vi "SUbvi double counter.vi"   [LabVIEW 2017]
uses:
  <vilib>/Platform/TimedLoop/XDataNode/timing_clust.ctl
  <vilib>/Platform/TimedLoop/XDataNode/nitl_modes.ctl
  <vilib>/Platform/TimedLoop/XDataNode/wakeup.ctl
  <vilib>/rvi/Emulation/niFpgaSctlEmulationGetInTimedLoop.vi
  <vilib>/rvi/Emulation/niFpgaEmulationReportErrorSimple.vi
  <vilib>/rvi/Emulation/niFpgaGetClockAttributes.vi
  <vilib>/rvi/Emulation/niFpgaCriticalErrorInLSC.vi
  <vilib>/rvi/eio/common/nirviEmuTemplateMethod_errors.vi
  <vilib>/Platform/TimedLoop/XDataNode/XDataNode.xnode
  <vilib>/eio/EIONode/EIONode.xnode
  <vilib>/Platform/TimedLoop/XDataNode/XDNodeRunTimeDep.lvlib
types:
  T1 = typedef "XDNodeRunTimeDep.lvlib/timing_clust.ctl" = cluster{"Expected End [f-1]":u64, "Actual End [f-1]":u64, "Finished Late? [f-1]":bool, "Expected End [i-1]":u64, "Actual End [i-1]":u64, "Finished Late? [i-1]":bool, "Expected Start [i]":u64, "Actual Start [i]":u64, "Expected Start [f]":u64, "Actual Start [f]":u64, "Source Name":string, "Structure Name":string, "Period":i64, "Deadline":i64, "Offset":i64, "Start":i64, "Priority":i32, "Timeout":i32, "Mode":T2, "Wakeup Reason":T3, "Error":errorcluster, "Source Type":string, "Secondary Source Type":string, "Global End Time":u64, "Global Start Time":u64, "Frame Duration":u64, "Iteration Duration":u64, "Assigned CPU":i32, "I/O Scan Engine Mode":u32}
  T2 = typedef "XDNodeRunTimeDep.lvlib/nitl_modes.ctl" = enum32{"No Change", "Process missed periods, maintain original phase", "Discard missed periods, maintain original phase", "Process missed periods, ignore original phase", "Discard missed periods, ignore original phase"}
  T3 = typedef "XDNodeRunTimeDep.lvlib/wakeup.ctl" = enum32{"Normal", "Aborted", "Asynchronous wakeup", "Timing source error", "Timed loop error", "Timeout"}
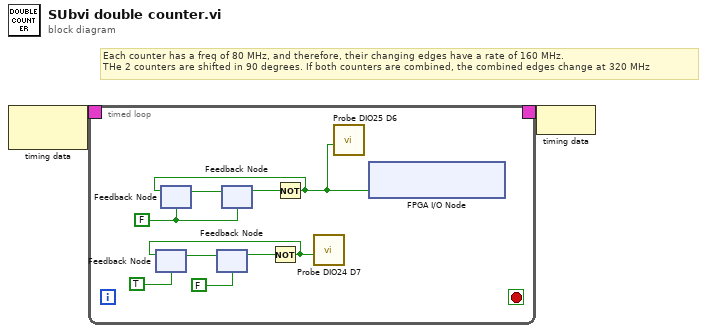
[diagram p0: block diagram]
diagram:
  # "Each counter has a freq of 80 MHz, and therefore, their changing edges have a rate of 160 MHz.\nTHe 2 counters are shifted in 90 degrees. If both counters are combined, the combined edges change at 320 MHz"
  n1 = node-c288() -> (w2:T1)  [unwired: 1 in]
  n2 = timed-loop {
    timing: w2 -> [_]
    timing-out: [_] -> w1
    stop <- _ stop-if-true
    w9 = FALSE
    n3 = feedback #1(TRUE) -> (w10:bool)
    n4 = feedback #2(w9) -> (w11:bool)
    n5 = feedback #3(FALSE) -> (w6:bool)
    n6 = feedback-in #3(w10) -> ()
    n7 = feedback #4(w9) -> (w8:bool)
    n8 = feedback-in #4(w11) -> ()
    n9 = Not(x=w6) -> (.not. x?=w3:bool)
    n10 = feedback-in #1(w3) -> ()
    n11 = Not(x=w8) -> (.not. x?=w4:bool)
    n12 = feedback-in #2(w4) -> ()
    n13 = call "Probe DIO24 D7.vi"("D7"=w3) -> ()  [unwired: 11 in]
    n14 = call "Probe DIO25 D6.vi"("D6"=w4) -> ()  [unwired: 11 in]
    n15 = xnode "FPGA I/O Node"("Connector0/DIO6"=w4) -> ()  [unwired: 1 in, 1 out]
  }
  n16 = node-c288(w1) -> ()
